vi "HEWH Read GEA Configuration.vi"() -> ()   [LabVIEW 2019]
uses:
  Utility/Save File/File Setup (Public)/Type Definition/Save File DOE File Path Control.ctl
  Utility/Save File/File Setup (Public)/Type Definition/Save File DOE Data Save Filepaths.ctl
  Utility/Save File/File Setup.lvlib
panel:
  out "appended array":T1[](array[typedef])
  in  "File Locations In":T1={"General Setup Paths"={"Calibration File Path"=path "", "DOE Capacity Path"=path "", "Data Folder Path"=path "", "RLT Backup Data Path"=path "", "Tool Base Path"=path "C:/GEA Water Heater Test Software", "General Startup Config Path"=path "", "File Save Previous Run Path"=path "", "File Save Configuration Data Path"=path ""}, "Data File Paths"={"Data File Path"=path "", "Debug File Path"=path "", "Bus Log Path"=path "", "Current"=path "", "Summary"=path ""}, "New Summary Created"=FALSE, "Check Location Interval (Second)"=0}
  in  "Populate Array?":bool=TRUE
  out "Board Index":i32[](array[numeric])
  out "Board ID":string[](array[string])
  in  "Array":path[](array[path])
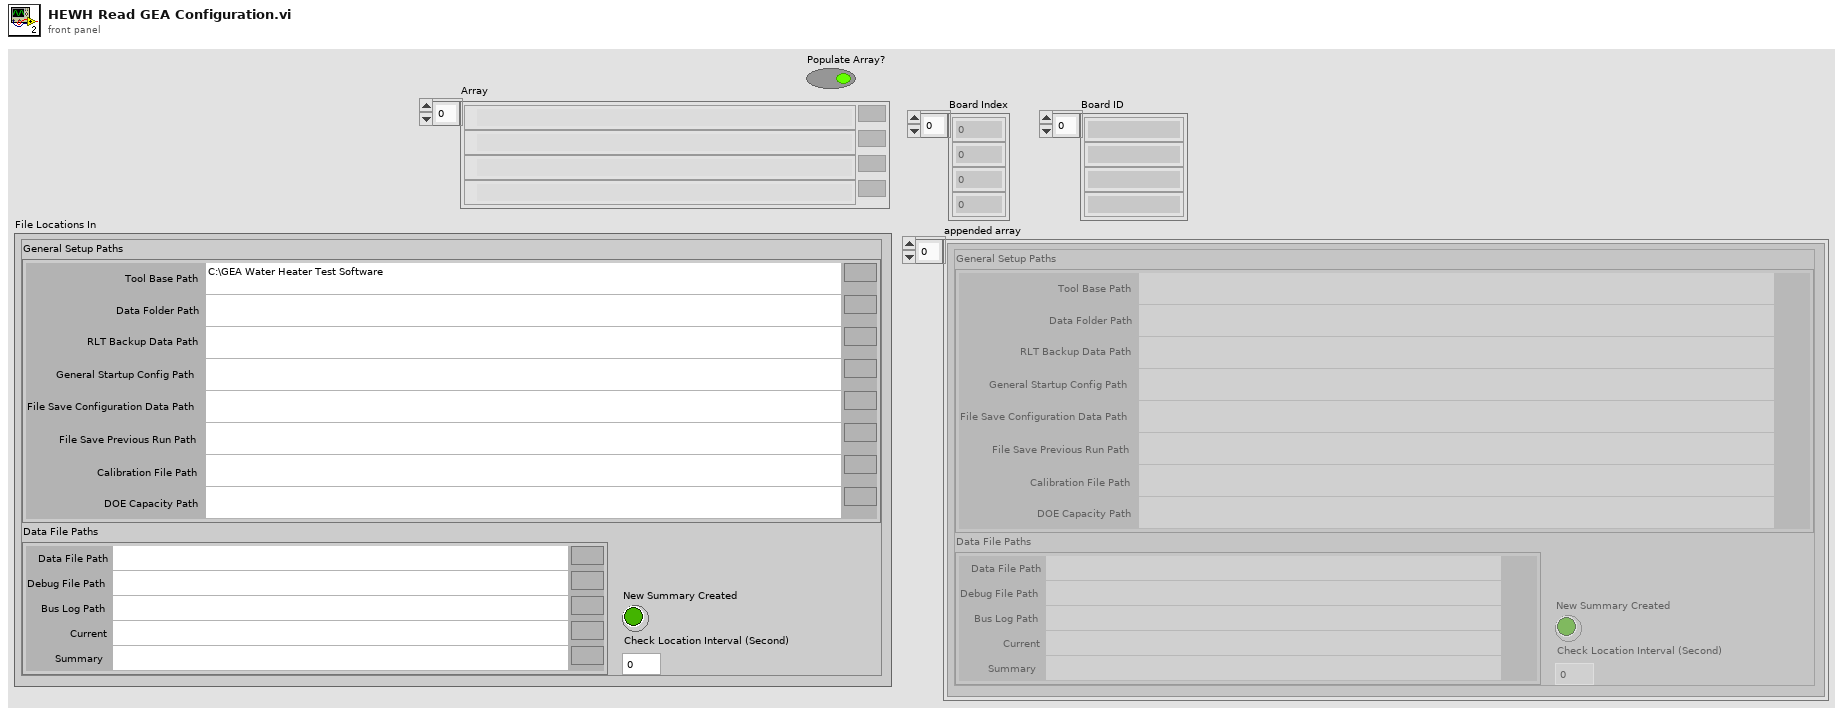
[diagram p1: front panel]
types:
  T1 = typedef "File Setup.lvlib/Save File DOE File Path Control.ctl" = cluster{"General Setup Paths":cluster{"Calibration File Path":path, "DOE Capacity Path":path, "Data Folder Path":path, "RLT Backup Data Path":path, "Tool Base Path":path, "General Startup Config Path":path, "File Save Previous Run Path":path, "File Save Configuration Data Path":path}, "Data File Paths":T2, "New Summary Created":bool, "Check Location Interval (Second)":i32}
  T2 = typedef "File Setup.lvlib/Save File DOE Data Save Filepaths.ctl" = cluster{"Data File Path":path, "Debug File Path":path, "Bus Log Path":path, "Current":path, "Summary":path}
  T3 = typedef "Save File.lvlib/Save File Washer.ctl" = cluster{"Appliance Details":T4, "Display Data (RLT)":T10}
  T4 = typedef "File Setup.lvlib/Save File DISH Dishwasher Details.ctl" = cluster{"FileVersionInfo":T5, "Dishwasher Info":cluster{"Open Cup Weight (gm):":dbl, "Auto Cup Weight (gm):":dbl, "Detergent-Dish:":string, "Inlet Temperature-Dish:":string, "Cycle Mode-Dish:":string, "Unit Control-Dish:":string, "Manufacturer-Dish:":string}, "Washer Info":cluster{"Hot Water Temperature (Fahrenheit):":string, "Cold Water Temperature (Fahrenheit):":string, "Capacity (cu.ft):":dbl, "Initial Cloth Weight:":dbl, "Cloth Lot:":i32, "Model Family:":string, "Program Name:":string, "Cycle Selection:":string, "Wash Temperature:":string, "Rinse Temperature:":string, "Load Size:":string}, "File Name Output Array":string[][], "Calibration Output Array":string[][], "Appliance Common":T6, "Water Heater":cluster{"Heating Mode:":string}, "Dryer":cluster{"Heat Setting:":T7, "Washer Water Temperature (60 ± 5°F):":u16, "Water Hardness (PPM):":u16, "Dryness Setting:":T7, "Dryer Type:":string, "Exhaust:":string, "Drying Cycle:":string, "Load Type:":string, "Nominal Load Weight":string, "Dryer Initial IMC Data":T8}}
  T5 = typedef "FileVersionInformation.ctl" = cluster{"FileVersion":string, "ProductName":string, "InternalName":string, "CompanyName":string, "LegalCopyright":string, "FileDescription":string}
  T6 = typedef "DOE Appliance Common.ctl" = cluster{"Engineer:":string, "Model Number:":string, "Serial Number:":string, "Comments:":string, "Station ID:":string, "Technician:":string, "TR Number:":string, "Lab ID:":string, "Voltage:":string, "Water Pressure (PSI):":string, "Test Date:":string, "Computer Name:":string, "IP Address:":string, "Ambient RH:":string, "Frequency:":string, "Build:":string, "Filename:":string, "Test Type:":string, "Load Run #:":i32, "Ambient Temperature (F):":string, "File Path:":path, "Cycles Per Year":u32}
  T7 = typedef "Custom Pallet String.ctl" = string
  T8 = typedef "DPT IMC Data.ctl" = cluster{"Measured IMC (lbs)":dbl, "Actual Initial RMC (%)":dbl, "RMC (Desired %)":dbl, "Bone Dry Wt(lbs)":dbl, "Tolerance(%)":dbl, "Actual Final RMC (%)":dbl, "CEF (lbf/kWh)":dbl, "Minimum Weight (lbf)":dbl, "Average Weight (lbf)":dbl, "Maximum Weight (lbf)":dbl, "Measured IMC In Range?":bool, "Moisture Reduction Factor":dbl, "Field Use Factor":dbl, "Empty Dryer Cold Weigth":dbl, "Energy Standard":T9, "Weight Cloth (lbs)":dbl, "Relative Moisture Content (%)":dbl, "Relative Moisture Content - Avg (%)":dbl}
  T9 = typedef "DOE Dryer Standard.ctl" = enum16{"D2-Automatic Dryer", "D2-Timer Dryer", "D1-Automatic Dryer", "D1-Timer Dryer", "Other"}
  T10 = typedef "Save File Appliance Display.ctl" = cluster{"Status Color":u32, "Serial Number Display":string, "Cycle Count Display":i32, "Station Label Display":string, "Current Run Start Time Display":dbl, "Board ID Display":string, "RPM Display":u32, "Current Display":dbl, "Current Path Display":path, "Saving Display":bool, "Unit Type Display":T11, "Total Time On Display":dbl, "UI Button":bool}
  T11 = typedef "Save File.lvlib/Save File Unit Type.ctl" = enum32{"", "Viper", "Hawk", "2015"}
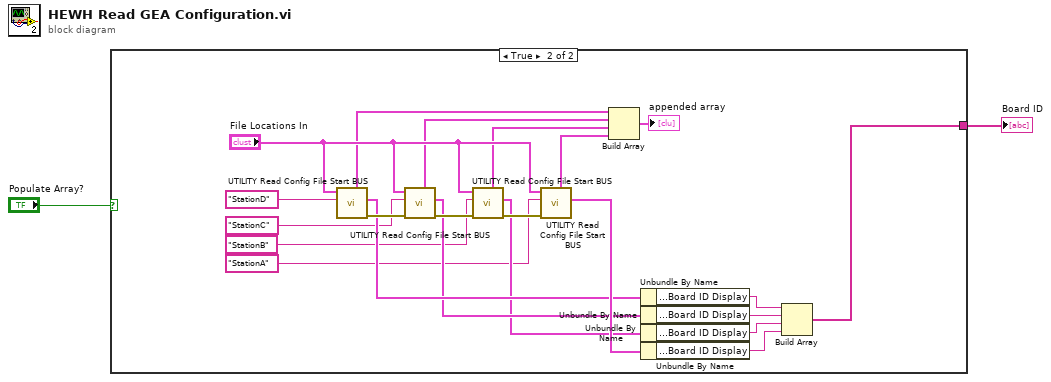
[diagram p0: block diagram]
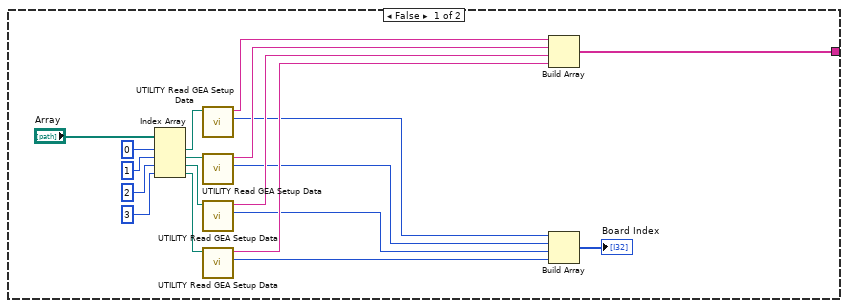
[diagram p2: hidden frame]
diagram:
  n1 = case shown="True" "Populate Array?" {
    tunnel: [w3 w26] -> w1
    frame False {
      n2 = Index Array(array="Array", index #1=0 ("index"), index #2=1 ("index"), index #3=2 ("index"), index #4=3 ("index")) -> (element #1=w16:path, element #2=w15:path, element #3=w14:path, element #4=w13:path)
      n3 = call "UTILITY Read GEA Setup Data.vi"("General Startup Config Path"=w16) -> ("Board Index"=w8:i32, "Board ID"=w12:string)  [unwired: 8 in, 1 out]
      n4 = call "UTILITY Read GEA Setup Data.vi"("General Startup Config Path"=w15) -> ("Board Index"=w7:i32, "Board ID"=w11:string)  [unwired: 8 in, 1 out]
      n5 = call "UTILITY Read GEA Setup Data.vi"("General Startup Config Path"=w14) -> ("Board Index"=w6:i32, "Board ID"=w10:string)  [unwired: 8 in, 1 out]
      n6 = call "UTILITY Read GEA Setup Data.vi"("General Startup Config Path"=w13) -> ("Board Index"=w5:i32, "Board ID"=w9:string)  [unwired: 8 in, 1 out]
      n7 = Build Array(w12, w11, w10, w9) -> (w3:string[])
      n8 = Build Array(w8, w7, w6, w5) -> (→"Board Index":i32[])
    }
    frame True {
      n9 = call "UTILITY Read Config File Start BUS.vi"("Station ID"="StationD", "File Locations In"="File Locations In") -> ("Error Out"=w37:errorcluster, "Main Washer Display Out"=w33:T3, "File Locations Out"=w42:T1)  [unwired: 6 in, 1 out]
      n10 = call "UTILITY Read Config File Start BUS.vi"("Error In"=w37, "Station ID"="StationC", "File Locations In"="File Locations In") -> ("Error Out"=w36:errorcluster, "Main Washer Display Out"=w32:T3, "File Locations Out"=w41:T1)  [unwired: 5 in, 1 out]
      n11 = call "UTILITY Read Config File Start BUS.vi"("Error In"=w36, "Station ID"="StationB", "File Locations In"="File Locations In") -> ("Error Out"=w35:errorcluster, "Main Washer Display Out"=w31:T3, "File Locations Out"=w40:T1)  [unwired: 5 in, 1 out]
      n12 = call "UTILITY Read Config File Start BUS.vi"("Error In"=w35, "Station ID"="StationA", "File Locations In"="File Locations In") -> ("Main Washer Display Out"=w34:T3, "File Locations Out"=w39:T1)  [unwired: 5 in, 2 out]
      n13 = Build Array(w42, w41, w40, w39) -> (→"appended array":T1[])
      n14 = Unbundle By Name(w33) -> ("Display Data (RLT).Board ID Display"=w30:string)
      n15 = Unbundle By Name(w32) -> ("Display Data (RLT).Board ID Display"=w29:string)
      n16 = Unbundle By Name(w31) -> ("Display Data (RLT).Board ID Display"=w28:string)
      n17 = Unbundle By Name(w34) -> ("Display Data (RLT).Board ID Display"=w27:string)
      n18 = Build Array(w30, w29, w28, w27) -> (w26:string[])
    }
  }
  "Board ID" <- w1
